vi "String, Timestamp, Integer, and Float to TDMS.vi"(0 "tdms file":refnum<k34>, 5 "Data Cluster Elements":variant[](array[variant]), 7 "Data Variant":variant, 9 "Group Name":string, 11 "error in (no error)":errorcluster) -> (4 "tdms file out":refnum<k34>, 15 "error out":errorcluster)   [LabVIEW 2023]
uses:
  <vilib>/Utility/Data Type/Type Definitions/Data Type.ctl
  <vilib>/Utility/Data Type/NI_Data Type.lvlib
panel:
  out "Troubleshoot - Types Found":T1[](array[typedef])
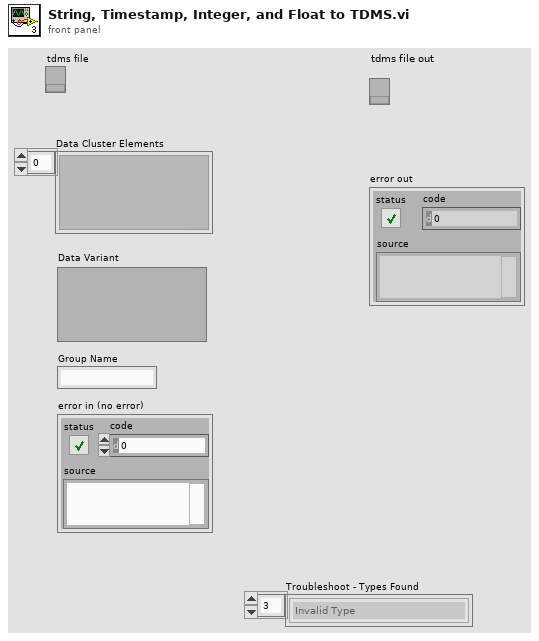
[diagram p1: front panel]
types:
  T1 = typedef "NI_Data Type.lvlib/Data Type.ctl" = enum8{"Invalid Type", "Void", "I8", "I16", "I32", "I64", "U8", "U16", "U32", "U64", "Single Float", "Double Float", "Extended Float", "Single Complex", "Double Complex", "Extended Complex", "Enum U8", "Enum U16", "Enum U32", "Enum U64", "Single Float With Unit", "Double Float With Unit", "Extended Float With Unit", "Single Complex with Unit", "Double Complex with Unit", "Extended Complex with Unit", "Boolean", "String", "Path", "Picture", "Tag", "Array", "Cluster", "Variant", "LV Variant", "Waveform", "Timestamp", "Digital Waveform", "Digital Data", "ExpressData", "Refnum", "External Data", "VI", "Poly VI", "LabVIEW Class Instance", "Fixed Point", "Set Collection", "Map Collection"}
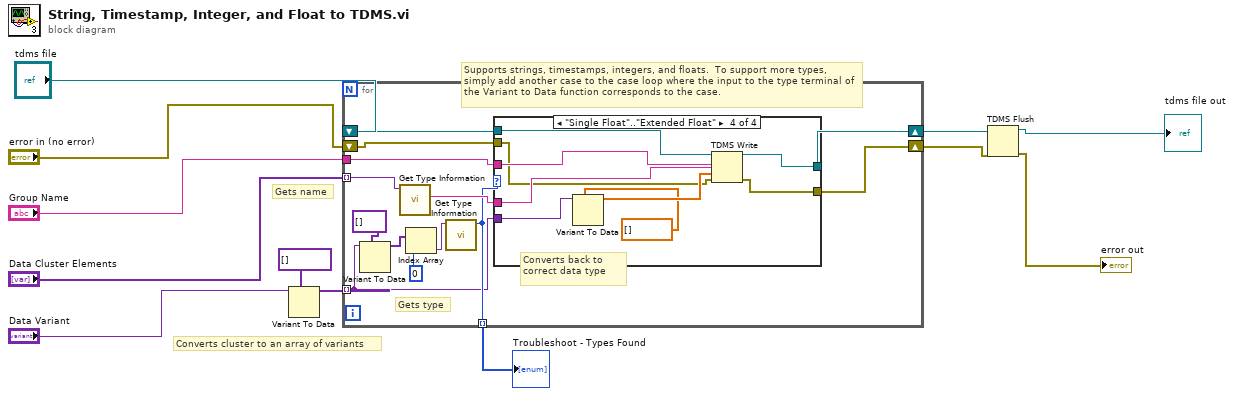
[diagram p0: block diagram]
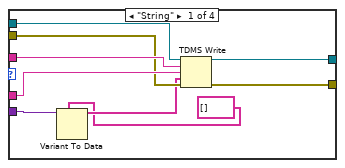
[diagram p2: hidden frame]
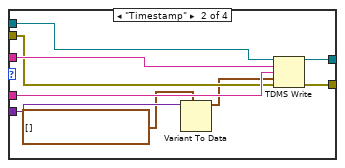
[diagram p3: hidden frame]
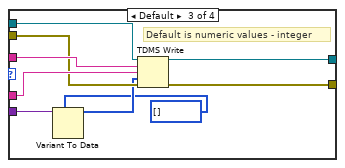
[diagram p4: hidden frame]
diagram:
  # "Gets name"
  # "Converts cluster to an array of variants"
  # "Supports strings, timestamps, integers, and floats.  To support more types, simply add another case to the case loop where the input to the type terminal of the Variant to Data function corresponds to the case."
  n1 = Variant To Data(type=variant[] [], Variant="Data Variant") -> (data=w12:variant[])  [unwired: 1 in, 1 out]
  n2 = for {
    tunnel: "Group Name" -> [w24]
    shift-right: [w22] -> w5
    shift-left: "tdms file" -> [w25]
    tunnel: w12 -> [w14] mode=indexing
    tunnel: "Data Cluster Elements" -> [w18] mode=indexing
    tunnel: [w20] -> w7 mode=indexing
    shift-right: [w21] -> w4
    shift-left: "error in (no error)" -> [w13]
    # "Gets type"
    # "Converts back to correct data type"
    n3 = Variant To Data(type=variant[] [], Variant=w14) -> (data=w16:variant[])  [unwired: 1 in, 1 out]
    n4 = call <vilib>:"Get Type Information.vi"("variant"=w18) -> ("name"=w23:string)  [unwired: 6 in, 4 out]
    n5 = Index Array(array=w16, index=0) -> (element=w19:variant)
    n6 = call <vilib>:"Get Type Information.vi"("variant"=w19) -> ("type"=w20:T1)  [unwired: 6 in, 4 out]
    n7 = case shown="\"Single Float\"..\"Extended Float\"" w20 {
      tunnel: w14 -> [w34 w39 w48 w61]
      tunnel: w25 -> [w33 w41 w49 w58]
      tunnel: w24 -> [w32 w43 w52 w60]
      tunnel: w23 -> [w31 w42 w50 w59]
      tunnel: [w30 w40 w51 w57] -> w22
      tunnel: w13 -> [w29 w38 w47 w53]
      tunnel: [w28 w37 w46 w56] -> w21
      frame "String" {
        n8 = Variant To Data(type=string[] [], Variant=w34) -> (data=w27:string[])  [unwired: 1 in, 1 out]
        n9 = TDMS Write(0:w33, 5:w32, 7:w31, 9:w27, 11:w29) -> (4:w30:refnum<k34>, 15:w28:errorcluster)  [unwired: 1 in, 2 out]
      }
      frame "Timestamp" {
        n10 = Variant To Data(type=timestamp[] [], Variant=w39) -> (data=w36:timestamp[])  [unwired: 1 in, 1 out]
        n11 = TDMS Write(0:w41, 5:w43, 7:w42, 9:w36, 11:w38) -> (4:w40:refnum<k34>, 15:w37:errorcluster)  [unwired: 1 in, 2 out]
      }
      frame Default {
        # "Default is numeric values - integer"
        n12 = Variant To Data(type=i32[] [], Variant=w48) -> (data=w45:i32[])  [unwired: 1 in, 1 out]
        n13 = TDMS Write(0:w49, 5:w52, 7:w50, 9:w45, 11:w47) -> (4:w51:refnum<k34>, 15:w46:errorcluster)  [unwired: 1 in, 2 out]
      }
      frame "Single Float".."Extended Float" {
        n14 = Variant To Data(type=dbl[] [], Variant=w61) -> (data=w55:dbl[])  [unwired: 1 in, 1 out]
        n15 = TDMS Write(0:w58, 5:w60, 7:w59, 9:w55, 11:w53) -> (4:w57:refnum<k34>, 15:w56:errorcluster)  [unwired: 1 in, 2 out]
      }
    }
  }
  "Troubleshoot - Types Found" <- w7
  n16 = TDMS Flush(4:w4, 7:w5) -> (0:→"error out":errorcluster, 3:→"tdms file out":refnum<k34>)
